vi "pinout-settings-get.vi"(8 "LabVIEW Web Service Request":refnum<class "Web Request.lvclass">) -> (16 "light_on_auto_mode":bool, 17 "ventilation_on_auto_mode":bool, 18 "ventilation_on_auto_treshold":u16, 19 "roof_sensor_data_pin":u8=4, 20 "main_light_pin":u8=8, 21 "main_fan_pin":u8=9, 22 "closed_roof_distance":dbl=3.0, 23 "roof_sensor_echo_pin":u8=5, 24 "main_light_on_auto_treshold":u16, 25 "outdoor_temp_pin":u8=2, 26 "light_on_threshold":u8=30, 27 "indoor_light_sensor_pin":u8=4)   [LabVIEW 2023]
uses:
  <vilib>/wsapi/Web Request.lvclass
  PinoutSettings.vi
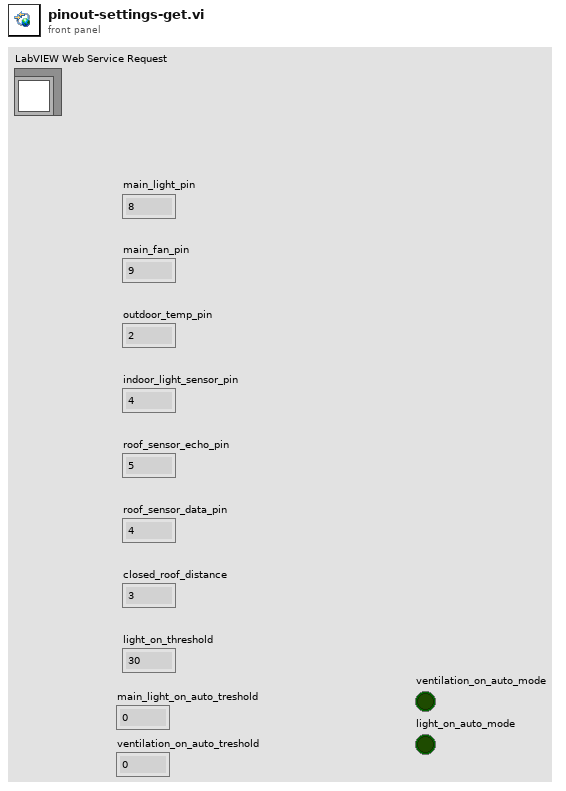
[diagram p1: front panel]
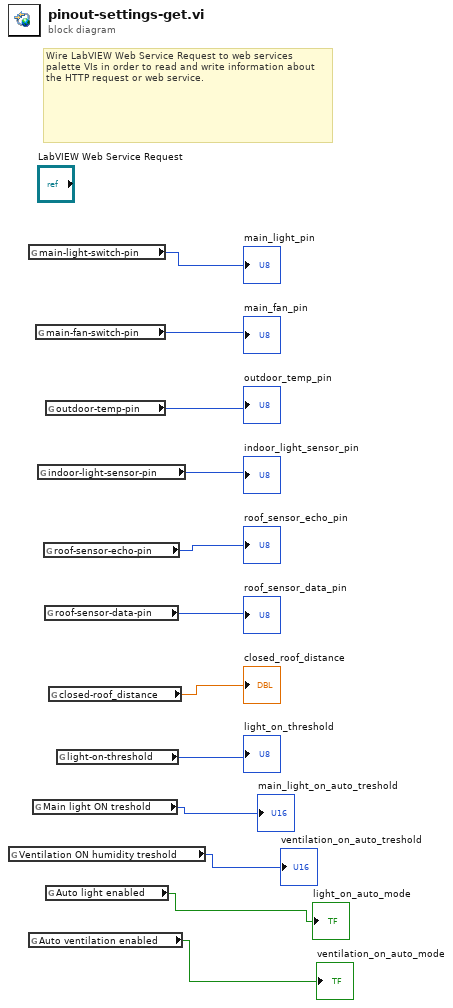
[diagram p0: block diagram]
diagram:
  # "Wire LabVIEW Web Service Request to web services palette VIs in order to read and write information about the HTTP request or web service."
  n1 = global read "PinoutSettings.vi" "Ventilation ON humidity treshold"() -> (→"ventilation_on_auto_treshold":u16)
  n2 = global read "PinoutSettings.vi" "main-light-switch-pin"() -> (→"main_light_pin":u8)
  n3 = global read "PinoutSettings.vi" "Auto ventilation enabled"() -> (→"ventilation_on_auto_mode":bool)
  n4 = global read "PinoutSettings.vi" "Main light ON treshold"() -> (→"main_light_on_auto_treshold":u16)
  n5 = global read "PinoutSettings.vi" "main-fan-switch-pin"() -> (→"main_fan_pin":u8)
  n6 = global read "PinoutSettings.vi" "indoor-light-sensor-pin"() -> (→"indoor_light_sensor_pin":u8)
  n7 = global read "PinoutSettings.vi" "roof-sensor-echo-pin"() -> (→"roof_sensor_echo_pin":u8)
  n8 = global read "PinoutSettings.vi" "roof-sensor-data-pin"() -> (→"roof_sensor_data_pin":u8)
  n9 = global read "PinoutSettings.vi" "outdoor-temp-pin"() -> (→"outdoor_temp_pin":u8)
  n10 = global read "PinoutSettings.vi" "Auto light enabled"() -> (→"light_on_auto_mode":bool)
  n11 = global read "PinoutSettings.vi" "closed-roof_distance"() -> (→"closed_roof_distance":dbl)
  n12 = global read "PinoutSettings.vi" "light-on-threshold"() -> (→"light_on_threshold":u8)
